vi "ROI entry-Dwell time switch.vi"(8 "error in (no error)":errorcluster, 11 "ROI Enum":T1) -> (0 "error out":errorcluster)   [LabVIEW 2013]
uses:
  Typedefs/ROI ID Enum.ctl
  Globals/gl_ROI Entry UI globals.vi
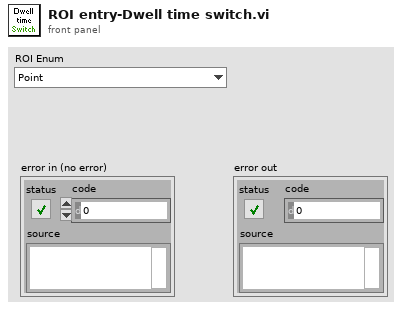
[diagram p1: front panel]
types:
  T1 = typedef "ROI ID Enum.ctl" = enum16{"Point", "MiniScan", "Comp. MiniScan", "Rectangle", "Comp. volume", "Arb. plane point"}
  T2 = typedef "ROI entry screen ctrl refs cluster.ctl" = cluster{"Done button":refnum<vi>, "Imaging button":refnum<vi>, "Acquisition button":refnum<vi>, "POI dwell time (us)":refnum<vi>, "Scan dwell time per pixel (us)":refnum<vi>, "# of planes":refnum<vi>, "Zoom":refnum<vi>, "Equal size":refnum<vi>, "Channel":refnum<vi>, "Image Display":refnum<vi>, "Z-Plane Selector":refnum<vi>, "Number of lines left":refnum<vi>, "Z-stack folder path":refnum<vi>, "POI Density":refnum<vi>, "Arb Plane Entry":refnum<vi>, "Whole plane":refnum<vi>, "Clear Last":refnum<vi>, "Clear All":refnum<vi>, "Trial Length (sec)":refnum<vi>, "Palette Type":refnum<vi>, "Intensity slider":refnum<vi>, "# POI":refnum<vi>, "Max Z Proj":refnum<vi>, "Zplane ind":refnum<vi>, "Wavelength (nm)":refnum<vi>, "Number of Trials":refnum<vi>, "Funct stim.trig.enable":refnum<vi>, "Funct stim.trig.delay (s)":refnum<vi>, "Line Mode":refnum<vi>, "Step size (µm)":refnum<vi>, "ROI move mode":refnum<vi>, "Cool-down time (s)":refnum<vi>, "Enable cool-down time":refnum<vi>, "Motor Z ind. (um)":refnum<vi>, "AOL Z ind. (um)":refnum<vi>}
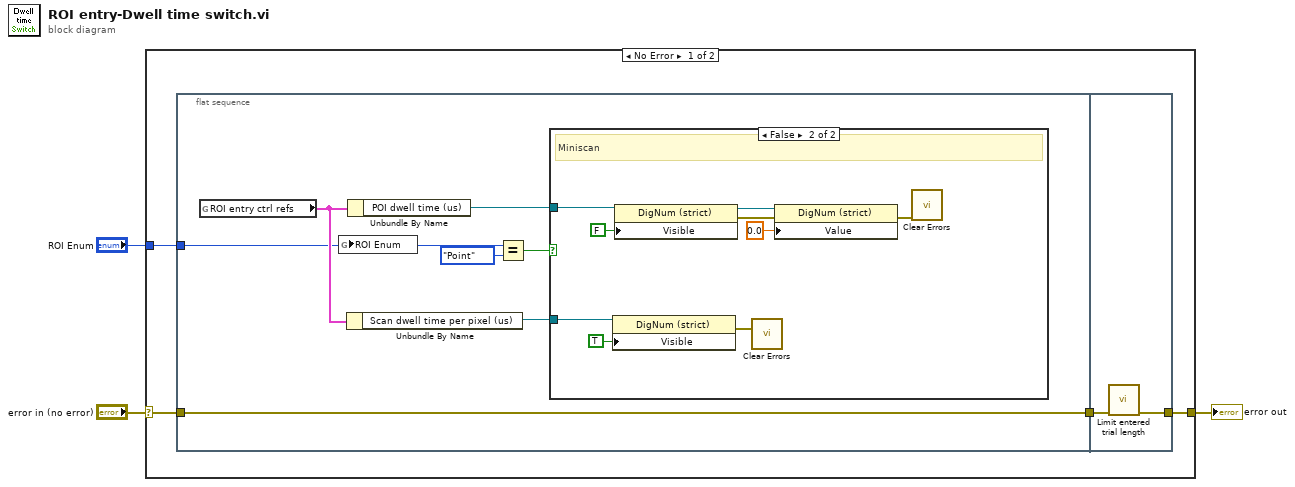
[diagram p0: block diagram]
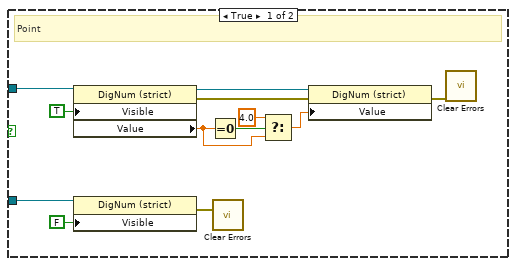
[diagram p2: hidden frame]
diagram:
  n1 = case shown="No Error" "error in (no error)" {
    selector: "error in (no error)" -> [w5 w38]
    tunnel: "ROI Enum" -> [w7 _]
    tunnel: [w4 w38] -> w1
    frame No Error {
      n2 = flat-sequence {
        tunnel: w7 -> [w9]
        tunnel: [w8] -> w6
        tunnel: w5 -> [w8]
        tunnel: w6 -> [w37]
        tunnel: [w36] -> w4
        frame #0 {
          n3 = global read "gl_ROI Entry UI globals.vi" "ROI entry ctrl refs"() -> (w11:T2)
          n4 = global write "gl_ROI Entry UI globals.vi" "ROI Enum"(w9) -> ()
          n5 = Unbundle By Name(w11) -> ("Scan dwell time per pixel (us)"=w13:refnum<vi>)
          n6 = Unbundle By Name(w11) -> ("POI dwell time (us)"=w12:refnum<vi>)
          n7 = Equal?(x=w9, y=ROI_ID_Enum."Point") -> (x = y?=w10:bool)
          n8 = case shown="False" w10 {
            tunnel: w13 -> [w26 w35]
            tunnel: w12 -> [w25 w34]
            frame True {
              # "Point"
              n9 = property on="Property Node" class="DigNum (strict)"(reference=w25, "Visible"=TRUE) -> (reference out=w20:refnum<vi>, error out=w21:errorcluster, "Value"=w15:dbl)  [unwired: 1 in]
              n10 = property on="Property Node" class="DigNum (strict)"(reference=w26, "Visible"=FALSE) -> (error out=w24:errorcluster)  [unwired: 1 in, 1 out]
              n11 = Equal To 0?(x=w15) -> (x = 0?=w18:bool)
              n12 = call <vilib>:"Clear Errors.vi"("error in (no error)"=w24) -> ()  [unwired: 6 in, 1 out]
              n13 = Select(t=4.0, s=w18, f=w15) -> (s? t:f=w16:dbl)
              n14 = property on="Property Node" class="DigNum (strict)"(reference=w20, error in=w21, "Value"=w16) -> (error out=w19:errorcluster)  [unwired: 1 out]
              n15 = call <vilib>:"Clear Errors.vi"("error in (no error)"=w19) -> ()  [unwired: 6 in, 1 out]
            }
            frame False {
              # "Miniscan"
              n16 = property on="Property Node" class="DigNum (strict)"(reference=w35, "Visible"=TRUE) -> (error out=w33:errorcluster)  [unwired: 1 in, 1 out]
              n17 = property on="Property Node" class="DigNum (strict)"(reference=w34, "Visible"=FALSE) -> (reference out=w29:refnum<vi>, error out=w30:errorcluster)  [unwired: 1 in]
              n18 = call <vilib>:"Clear Errors.vi"("error in (no error)"=w33) -> ()  [unwired: 6 in, 1 out]
              n19 = property on="Property Node" class="DigNum (strict)"(reference=w29, error in=w30, "Value"=0.0) -> (error out=w28:errorcluster)  [unwired: 1 out]
              n20 = call <vilib>:"Clear Errors.vi"("error in (no error)"=w28) -> ()  [unwired: 6 in, 1 out]
            }
          }
        }
        frame #1 {
          n21 = call "Limit entered trial length.vi"("error in (no error)"=w37) -> ("error out"=w36:errorcluster)  [unwired: 10 in]
        }
      }
    }
    frame Error {
    }
  }
  "error out" <- w1
